vi "HovaCAL_Interface_SetFlow.vi"(8 "error in (no error)":errorcluster caption="Fehler (Eingang, kein Fehler)", 10 "sofort":bool=TRUE, 11 "total flow setpoint":dbl) -> (0 "error out":errorcluster caption="Fehler (Ausgang)")   [LabVIEW 2020, in "Linearisierung v2.lvlib" / "Gasteiler.lvlib" / "HovaCAL_Interface.lvlib" / "Kommunikation.lvlib"]
uses:
  Kommunikation.lvlib
  Aktion_FGV_HovaCAL_Interface_SetData.ctl
  Aktion_FGV_HovaCAL_Interface_Kommandos.ctl
  Aktion_FGV_HovaCAL_Interface_Kommunikation.ctl
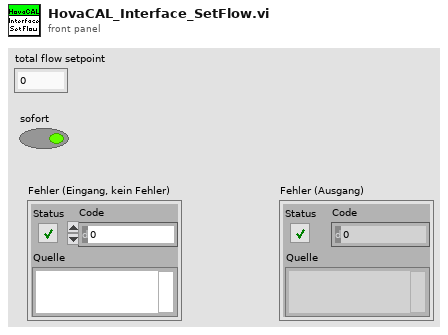
[diagram p1: front panel]
types:
  T1 = typedef "Linearisierung v2.lvlib/Gasteiler.lvlib/HovaCAL_Interface.lvlib/Kommunikation.lvlib/Aktion_FGV_HovaCAL_Interface_SetData.ctl" = enum16{"lesen", "Konzentrationen", "Pumpen Parameter", "Pumpe Konzentration", "Pumpe run", "Temperaturen", "Fluss", "Limits", "init"}
  T2 = typedef "Linearisierung v2.lvlib/Gasteiler.lvlib/HovaCAL_Interface.lvlib/Kommunikation.lvlib/Aktion_FGV_HovaCAL_Interface_Kommandos.ctl" = enum16{"lesen", "verarbeiten", "hinzufügen", "on top", "init", "sammeln", "freigeben", "connected"}
  T3 = typedef "Linearisierung v2.lvlib/Gasteiler.lvlib/HovaCAL_Interface.lvlib/Kommunikation.lvlib/Aktion_FGV_HovaCAL_Interface_Kommunikation.ctl" = enum16{"Initialisieren", "Set Konzentrationen", "Set Gase", "Set Limits", "Get Dynamische Werte", "Beenden", "Com ändern", "Get Gase init", "Pause", "Get Gasteiler Infos", "Get MFC Infos", "Set Pumpen Parameter", "Set Pumpe Konzenration", "Set Pumpe run", "Set Temperaturen", "Set Fluss", "Get Gase", "Get Limits", "Get Dynamische Werte 1", "Get Dynamische Werte 2"}
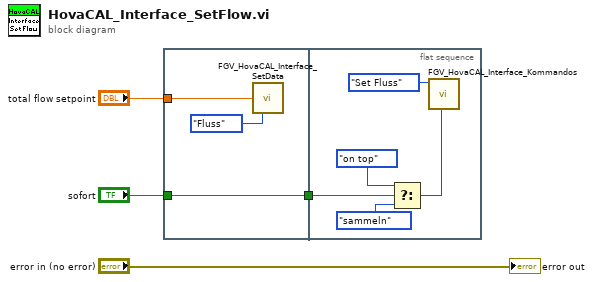
[diagram p0: block diagram]
diagram:
  n1 = flat-sequence {
    tunnel: "total flow setpoint" -> [w6]
    tunnel: [w5] -> w3
    tunnel: "sofort" -> [w5]
    tunnel: w3 -> [w11]
    frame #0 {
      n2 = call "FGV_HovaCAL_Interface_SetData.vi"("total flow setpoint in"=w6, "Aktion"=Aktion_FGV_HovaCAL_Interface_SetData."Fluss") -> ()  [unwired: 7 in, 7 out]
    }
    frame #1 {
      n3 = Select(t=Aktion_FGV_HovaCAL_Interface_Kommandos."on top" ("Aktion"), s=w11, f=Aktion_FGV_HovaCAL_Interface_Kommandos."sammeln") -> (s? t:f=w9:T2)
      n4 = call "FGV_HovaCAL_Interface_Kommandos.vi"("Aktion"=w9, "Kommando in"=Aktion_FGV_HovaCAL_Interface_Kommunikation."Set Fluss") -> ()  [unwired: 3 in, 6 out]
    }
  }
  "error out" <- "error in (no error)"
